vi "gui_formatTable.vi"() -> (0 "column size":u32, 1 "column header":string[](array[string])=["DC Voltage", "DC Current", "DC Power", "AC Voltage", "AC Current", "AC Power", "Interter Effiency", "Torque", "Speed", "Output Power", "Overall Effiency"], 2 "row size":u32, 3 "row header":string[](array[string])=["DC Voltage", "DC Current", "DC Power", "AC Voltage", "AC Current", "AC Power", "Interter Effiency", "Torque", "Speed", "Output Power", "Overall Effiency"])   [LabVIEW 2019]
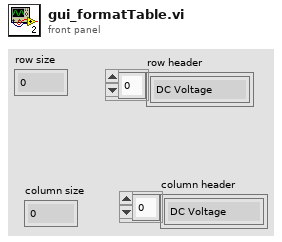
[diagram p1: front panel]
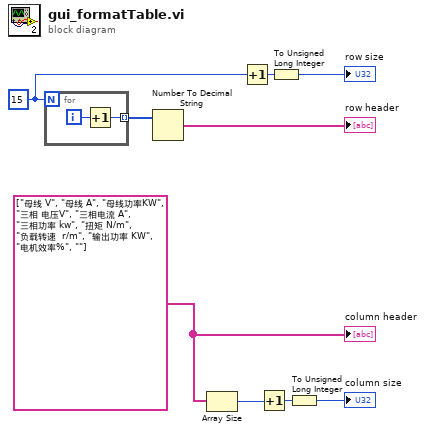
[diagram p0: block diagram]
diagram:
  w5 = 15
  w9 = string[] ["母线 V", "母线 A", "母线功率KW", "三相 电压V", "三相电流 A", "三相功率 kw", "扭矩 N/m", "负载转速  r/m", "输出功率 KW", "电机效率%", ""]
  n1 = for {
    N: w5 -> [_]
    tunnel: [w10] -> w6 mode=indexing
    i -> [w11]
    n2 = Increment(x=w11) -> (x+1=w10:i32)
  }
  n3 = Number To Decimal String(number=w6) -> (decimal integer string=→"row header":string[])  [unwired: 1 in]
  n4 = Array Size(array=w9) -> (size(s)=w8:i32)
  n5 = Increment(x=w5) -> (x+1=w3:i32)
  n6 = Increment(x=w8) -> (x+1=w7:i32)
  n7 = To Unsigned Long Integer(number=w3) -> (unsigned 32bit integer=→"row size":u32)
  n8 = To Unsigned Long Integer(number=w7) -> (unsigned 32bit integer=→"column size":u32)
  "column header" <- w9
